vi "Run.vi"(8 "error in (no error)":errorcluster, 11 "Tread in":refnum<class "Tread.lvclass">) -> (0 "error out":errorcluster, 3 "Tread out":refnum<class "Tread.lvclass">)   [LabVIEW 2020, in "Tread.lvclass"]
uses:
  Tread.lvclass
  bno055/BNO055/BNO055/Calibration Status.ctl
  bno055/BNO055/BNO055/Euler Angles.ctl
  nmea/nmea/nmea/Full Data.ctl
  nmea/nmea/nmea/Fix.ctl
  nmea/nmea/nmea/Velocity.ctl
  nmea/nmea/nmea/DOP.ctl
  nmea/nmea/nmea/Satellite.ctl
  nmea/nmea/nmea/Fix Type.ctl
  nmea/nmea/nmea/Fix Mode.ctl
  Tread.lvclass/Tread.ctl
  bno055/BNO055/BNO055/BNO055.lvclass
  nmea/nmea/VISA GPS/VISA GPS.lvclass
  nmea/nmea/nmea/nmea.lvclass
panel:
  out "Full Data":T1 {"Fix"."Longitude" format="%_16f"; "Fix"."Latitude" format="%_16f"}
  out "Euler Angles":T8
  out "Calibration Status":T9
  in  "stop":bool
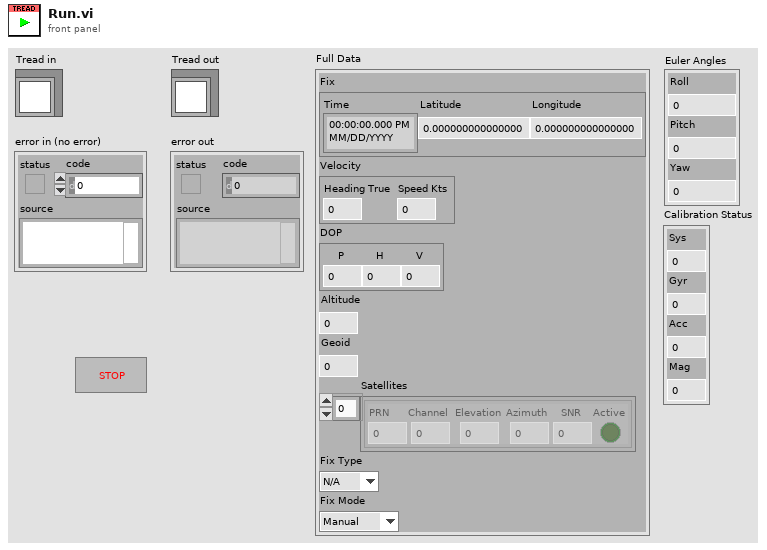
[diagram p1: front panel]
types:
  T1 = typedef "nmea.lvlib/nmea.lvclass/Full Data.ctl" = cluster{"Fix":T2, "Velocity":T3, "DOP":T4, "Altitude":dbl, "Geoid":dbl, "Satellites":T5[], "Fix Type":T6, "Fix Mode":T7}
  T2 = typedef "nmea.lvlib/nmea.lvclass/Fix.ctl" = cluster{"Time":timestamp, "Latitude":dbl, "Longitude":dbl}
  T3 = typedef "nmea.lvlib/nmea.lvclass/Velocity.ctl" = cluster{"Heading True":dbl, "Speed Kts":dbl}
  T4 = typedef "nmea.lvlib/nmea.lvclass/DOP.ctl" = cluster{"P":dbl, "H":dbl, "V":dbl}
  T5 = typedef "nmea.lvlib/nmea.lvclass/Satellite.ctl" = cluster{"PRN":u8, "Channel":u8, "Elevation":u8, "Azimuth":u16, "SNR":u8, "Active":bool}
  T6 = typedef "nmea.lvlib/nmea.lvclass/Fix Type.ctl" = enum16{"N/A", "None", "2D", "3D"}
  T7 = typedef "nmea.lvlib/nmea.lvclass/Fix Mode.ctl" = enum16{"Manual", "Auto 2/3D"}
  T8 = typedef "BNO055.lvlib/BNO055.lvclass/Euler Angles.ctl" = cluster{"Roll":dbl, "Pitch":dbl, "Yaw":dbl}
  T9 = typedef "BNO055.lvlib/BNO055.lvclass/Calibration Status.ctl" = cluster{"Sys":u8, "Gyr":u8, "Acc":u8, "Mag":u8}
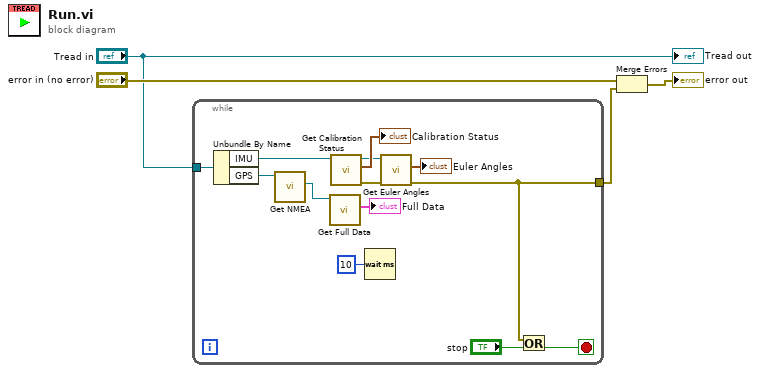
[diagram p0: block diagram]
diagram:
  n1 = while {
    tunnel: "Tread in" -> [w17]
    tunnel: [w5] -> w1
    stop <- w6 stop-if-true
    n2 = Unbundle By Name(w17) -> ("IMU"=w15:refnum<class "BNO055.lvclass">, "GPS"=w11:refnum<class "VISA GPS.lvclass">)
    n3 = call "Get NMEA.vi"("VISA GPS in"=w11) -> ("NMEA"=w10:refnum<class "nmea.lvclass">)  [unwired: 8 in, 2 out]
    n4 = call "Get Full Data.vi"("nmea in"=w10) -> ("Full Data"=→"Full Data":T1)  [unwired: 8 in, 2 out]
    n5 = call "Get Calibration Status.vi"("BNO055 in"=w15) -> ("error out"=w7:errorcluster, "Calibration Status"=→"Calibration Status":T9, "BNO055 out"=w13:refnum<class "BNO055.lvclass">)  [unwired: 8 in]
    n6 = Wait (ms)(milliseconds to wait=u32 10) -> ()  [unwired: 1 out]
    n7 = call "Get Euler Angles.vi"("error in (no error)"=w7, "BNO055 in"=w13) -> ("error out"=w5:errorcluster, "Euler Angles"=→"Euler Angles":T8)  [unwired: 7 in, 1 out]
    n8 = Or(x=w5, y="stop") -> (x .or. y?=w6:bool)
  }
  n9 = Merge Errors("error in (no error)", w1) -> (→"error out":errorcluster)
  "Tread out" <- "Tread in"
